vi "EOL CAN_Read HW level.vi"(8 "error in (no error)":errorcluster, 10 "Read Session in":refnum<k21>, 11 "Write Session in":refnum<k21>) -> (0 "error out":errorcluster, 1 "HW level":string, 2 "Response Good?":bool, 3 "TxRx Data":string[][](array[string]))   [LabVIEW 2018]
uses:
  <vilib>/xnet/xnet.llb/XNET Frame CAN.ctl
  <vilib>/xnet/xnet.llb/XNET Frame Type CAN.ctl
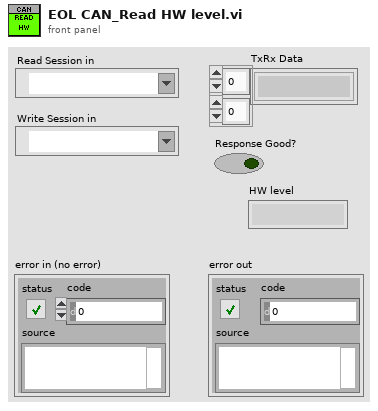
[diagram p1: front panel]
types:
  T1 = typedef "XNET Frame CAN.ctl" = cluster{"timestamp":timestamp, "payload":u8[], "identifier":u32, "type":T2, "extended?":bool, "echo?":bool}
  T2 = typedef "XNET Frame Type CAN.ctl" = u8
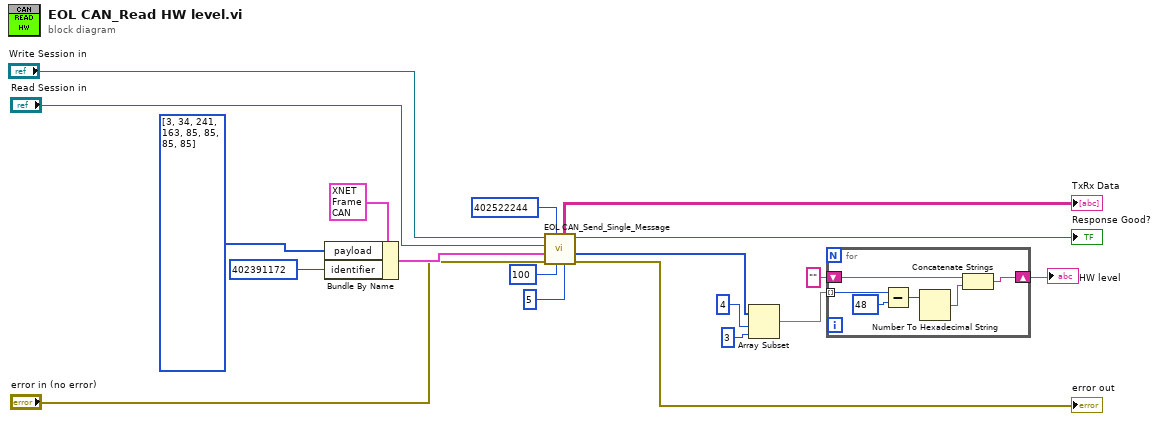
[diagram p0: block diagram]
diagram:
  n1 = Bundle By Name(cluster=T1 {"timestamp"=timestamp(0 s since 1904-01-01), "payload"=[2, 39, 3, 85, 85, 85, 85, 85], "identifier"=402391172, "type"=0, "extended?"=TRUE, "echo?"=FALSE} ("Tx CAN frame"), "payload"=u8[] [3, 34, 241, 163, 85, 85, 85, 85], "identifier"=u32 402391172) -> (w17:T1)
  n2 = call <userlib>:"EOL CAN_Send_Single_Message.vi"("Retries"=5, "Msg Wait Time"=u32 100, "Rx Arbitration Id"=u32 402522244, "Error in"="error in (no error)", "Tx CAN frame"=w17, "Read Session in"="Read Session in", "Write Session in"="Write Session in") -> ("Error out"=→"error out":errorcluster, "Rx Message"=w4:u8[], "Response Good?"=→"Response Good?":bool, "TxRx Data"=→"TxRx Data":string[][])  [unwired: 1 out]
  n3 = Array Subset(array=w4, index=4, length=3) -> (w2:u8[])
  n4 = for {
    tunnel: w2 -> [w21] mode=indexing
    shift-right: [w23] -> w1
    shift-left: "" -> [w25]
    n5 = Subtract(x=w21, y=u8 48) -> (x-y=w20:u8)
    n6 = Number To Hexadecimal String(2:w20) -> (0:w24:string)  [unwired: 1 in]
    n7 = Concatenate Strings(w25, w24) -> (w23:string)
  }
  "HW level" <- w1
